vi "Step Update Map - Description Updated.vi"(10 "New Description":string, 11 "Step Number":i32) -> (3 "Step Update Map out":T1(c390))   [LabVIEW 2020, in "Output Sequencer.lvlib" / "Settings UI.lvclass"]
uses:
  Settings UI.lvclass
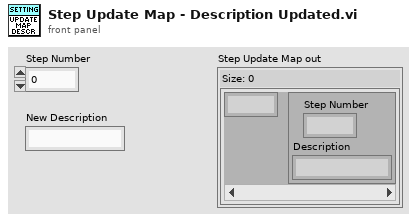
[diagram p1: front panel]
types:
  T1 = map{i32, cluster{"Step Number":i32, "Description":string}}
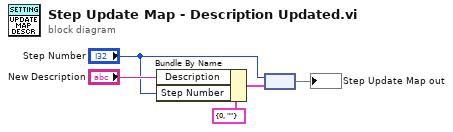
[diagram p0: block diagram]
diagram:
  n1 = Bundle By Name(cluster=cluster{"Step Number":i32, "Description":string} {"Step Number"=0, "Description"=""} ("New Settings"), "Description"="New Description", "Step Number"="Step Number") -> (w3:cluster{"Step Number":i32, "Description":string})
  n2 = node("Step Number", w3) -> (→"Step Update Map out":T1)
